vi "V-Meter Configure (2000).vi"(8 "error in (no error)":errorcluster, 11 "VISA resource name in":refnum<visa-resource-name>) -> (0 "error out":errorcluster, 3 "VISA resource name out":refnum<visa-resource-name>)   [LabVIEW 2016, in "Hall Effect Library.lvlib"]
uses:
  Hall Effect Library.lvlib
  Global Variables/Test Settings.vi
  <instrlib>/Keithley 2000/Public/Configure/Configure DC Volts.vi
  <instrlib>/Keithley 2000/Keithley 2000.lvlib
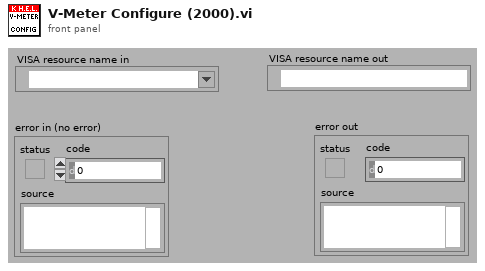
[diagram p1: front panel]
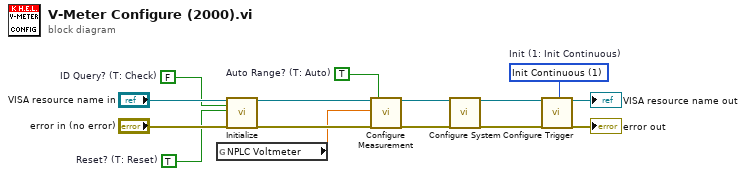
[diagram p0: block diagram]
diagram:
  w6 = i16 1 items=["Don't Init"=-1, "Init Single"=0, "Init Continuous"=1]  # Init (1: Init Continuous)
  w9 = TRUE  # Auto Range? (T: Auto)
  w12 = FALSE  # ID Query? (T: Check)
  w13 = TRUE  # Reset? (T: Reset)
  n1 = global read "Test Settings.vi" "NPLC Voltmeter"() -> (w1:dbl)
  n2 = call <instrlib>:"Initialize.vi"("VISA resource name"="VISA resource name in", "ID Query? (T: Check)"=w12, "Reset? (T: Reset)"=w13, "error in (no error)"="error in (no error)") -> ("VISA resource name out"=w10:refnum<visa-resource-name>, "error out"=w11:errorcluster)  [unwired: 14 out]
  n3 = call-poly <instrlib>:"Configure Measurement.vi"("VISA resource name"=w10, "Power Line Cycles (1.00)"=w1, "error in (no error)"=w11, "Auto Range? (T: Auto)"=w9) -> ("VISA resource name out"=w3:refnum<visa-resource-name>, "error out"=w2:errorcluster)  [unwired: 6 in, 8 out]
  n4 = call <instrlib>:"Configure System.vi"("VISA resource name"=w3, "error in (no error)"=w2) -> ("VISA resource name out"=w4:refnum<visa-resource-name>, "error out"=w5:errorcluster)  [unwired: 2 in, 14 out]
  n5 = call <instrlib>:"Configure Trigger.vi"("VISA resource name"=w4, "error in (no error)"=w5, "Init (1: Init Continuous)"=w6) -> ("VISA resource name out"=→"VISA resource name out":refnum<visa-resource-name>, "error out"=→"error out":errorcluster)  [unwired: 6 in, 9 out]
